vi "Collate_graphs.vi"(4 "R values":dbl[](array[numeric]), 5 "rho0":dbl[](array[numeric]), 6 "rho-":dbl[](array[numeric]), 7 "rho+":dbl[](array[numeric]), 9 "AFP Range":cluster{"Numeric":i32, "Numeric 2":i32}, 10 "RF Range 2":cluster{"Numeric":i32, "Numeric 2":i32}, 11 "RF Range 1":cluster{"Numeric":i32, "Numeric 2":i32}) -> (2 "Q Graph":cluster{"Array":dbl[], "Array 2":dbl[]}, 3 "P Graph and Intensities and RF":cluster{"Array":dbl[], "Array":dbl[]}[](array[cluster]))   [LabVIEW 2018]
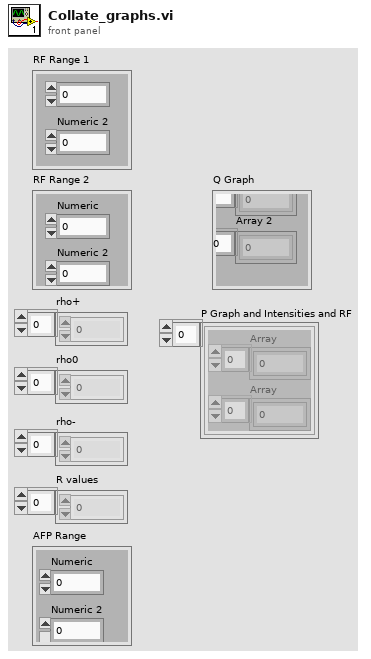
[diagram p1: front panel]
types:
  T1 = cluster{"R values":dbl[], "Output Array":dbl[]}[]
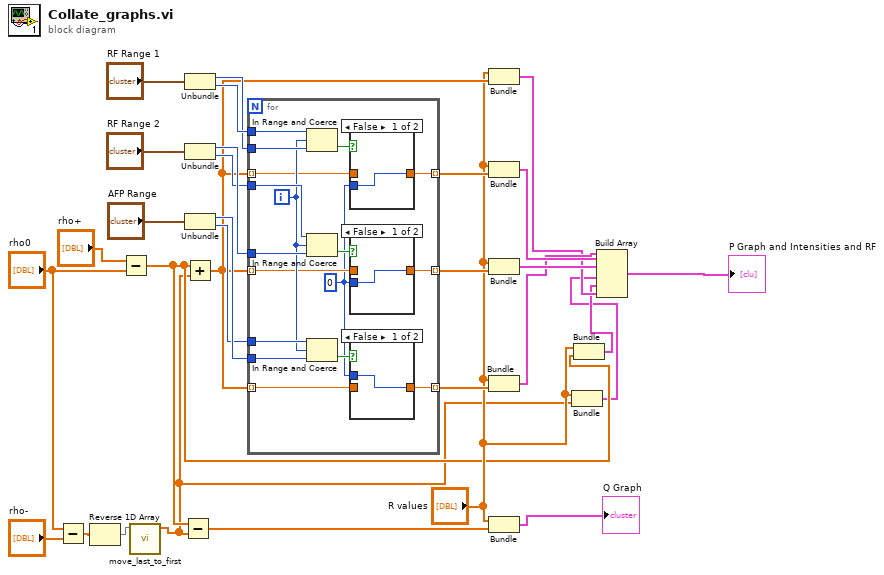
[diagram p0: block diagram]
diagram:
  n1 = Subtract(x="rho0", y="rho-") -> (x-y=w27:dbl[])
  n2 = Reverse 1D Array(array=w27) -> (reversed array=w2:dbl[])
  n3 = Subtract(x="rho+", y="rho0") -> (x-y=w5:dbl[])
  n4 = call "move_last_to_first.vi"("Input array"=w2) -> ("Output Array"=w1:dbl[])  [unwired: 10 in]
  n5 = Subtract(x=w5, y=w1) -> (x-y=w13:dbl[])
  n6 = Unbundle("RF Range 1") -> ("Numeric"=w22:i32, "Numeric 2"=w23:i32)
  n7 = Unbundle("RF Range 2") -> ("Numeric"=w21:i32, "Numeric 2"=w20:i32)
  n8 = Unbundle("AFP Range") -> ("Numeric"=w19:i32, "Numeric 2"=w18:i32)
  n9 = Add(x=w5, y=w1) -> (x+y=w14:dbl[])
  n10 = for {
    tunnel: w23 -> [w47]
    tunnel: w22 -> [w46]
    tunnel: w21 -> [w42]
    tunnel: w20 -> [w41]
    tunnel: w19 -> [w40]
    tunnel: w18 -> [w39]
    tunnel: w14 -> [w37] mode=indexing
    tunnel: w14 -> [w36] mode=indexing
    tunnel: w14 -> [w35] mode=indexing
    tunnel: [w34] -> w17 mode=indexing
    tunnel: [w33] -> w15 mode=indexing
    tunnel: [w32] -> w16 mode=indexing
    i -> [w38]
    w31 = 0
    n11 = In Range and Coerce(upper limit=w47, x=w38, lower limit=w46) -> (In Range?=w43:bool)  [unwired: 1 out]
    n12 = In Range and Coerce(upper limit=w41, x=w38, lower limit=w42) -> (In Range?=w44:bool)  [unwired: 1 out]
    n13 = In Range and Coerce(upper limit=w39, x=w38, lower limit=w40) -> (In Range?=w45:bool)  [unwired: 1 out]
    n14 = case shown="False" w43 {
      tunnel: w37 -> [_ w53]
      tunnel: [w52 w53] -> w34
      tunnel: w31 -> [w52 _]
      frame False {
      }
      frame True {
      }
    }
    n15 = case shown="False" w44 {
      tunnel: w36 -> [_ w51]
      tunnel: [w50 w51] -> w33
      tunnel: w31 -> [w50 _]
      frame False {
      }
      frame True {
      }
    }
    n16 = case shown="False" w45 {
      tunnel: w35 -> [_ w49]
      tunnel: [w48 w49] -> w32
      tunnel: w31 -> [w48 _]
      frame False {
      }
      frame True {
      }
    }
  }
  n17 = Bundle("R values"="R values", w14) -> (w7:cluster{"R values":dbl[], dbl[]})  [unwired: 1 in]
  n18 = Bundle("R values"="R values", w17) -> (w12:cluster{"R values":dbl[], dbl[]})  [unwired: 1 in]
  n19 = Bundle("R values"="R values", w15) -> (w11:cluster{"R values":dbl[], dbl[]})  [unwired: 1 in]
  n20 = Bundle("R values"="R values", w16) -> (w8:cluster{"R values":dbl[], dbl[]})  [unwired: 1 in]
  n21 = Bundle("R values"="R values", w13) -> (→"Q Graph":cluster{"R values":dbl[], dbl[]})  [unwired: 1 in]
  n22 = Bundle("R values"="R values", "Output Array"=w1) -> (w3:cluster{"R values":dbl[], "Output Array":dbl[]})  [unwired: 1 in]
  n23 = Bundle("R values"="R values", w5) -> (w4:cluster{"R values":dbl[], dbl[]})  [unwired: 1 in]
  n24 = Build Array(w8, w12, w11, w3, w4, w7) -> (→"P Graph and Intensities and RF":T1)
